vi "SetFurniture.vi"(8 "error in (no error)":errorcluster, 10 "Furniture":refnum<class "Furniture.lvclass">[](array[class]), 11 "RoomB in":refnum<class "RoomB.lvclass">) -> (0 "error out":errorcluster, 3 "RoomB out":refnum<class "RoomB.lvclass">)   [LabVIEW 2019, in "RoomB.lvclass"]
uses:
  RoomB.lvclass
  Room.lvclass
  Furniture.lvclass
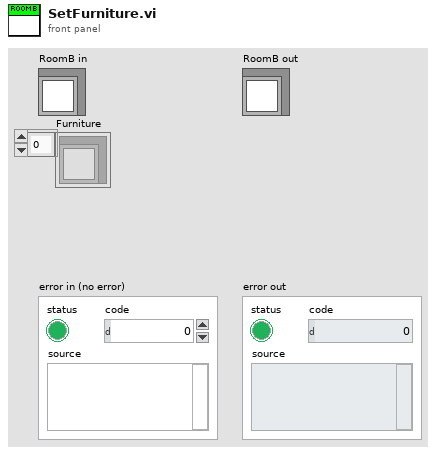
[diagram p1: front panel]
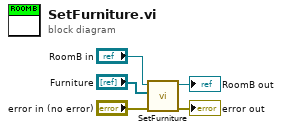
[diagram p0: block diagram]
diagram:
  n1 = call-parent "SetFurniture.vi"("error in (no error)"="error in (no error)", "Furniture"="Furniture", "Room in"="RoomB in") -> ("error out"=→"error out":errorcluster, "Room out"=→"RoomB out":refnum<class "RoomB.lvclass">)  [unwired: 7 in]
